vi "add_alignment_text.vi"(4 "Font, Size & Style":T1, 6 "Color":u32, 11 "image in":T2) -> (3 "image out":T2)   [LabVIEW 2011]
uses:
  <vilib>/vision/Image Controls.llb/IMAQ Image.ctl
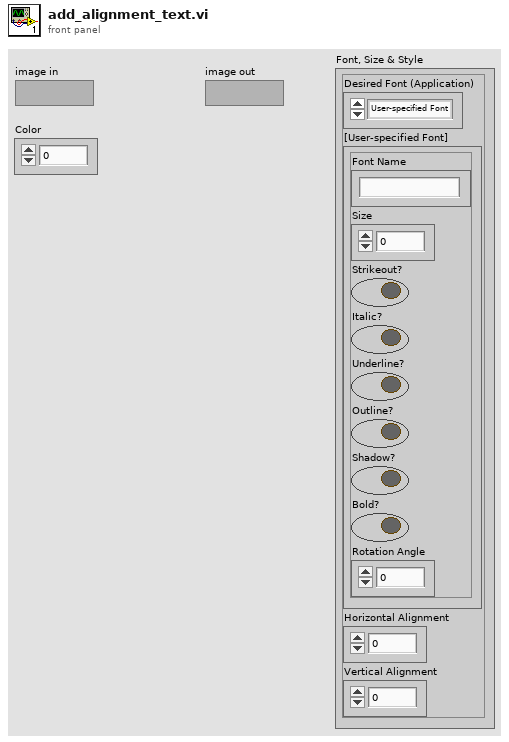
[diagram p1: front panel]
types:
  T1 = cluster{"Desired Font (Application)":enum16{"User-specified Font", "Application Font", "System Font", "Dialog Font"}, "[User-specified Font]":cluster{"Font Name":string, "Size":i16, "Strikeout?":bool, "Italic?":bool, "Underline?":bool, "Outline?":bool, "Shadow?":bool, "Bold?":bool, "Rotation Angle":dbl}, "Horizontal Alignment":i16, "Vertical Alignment":i16}
  T2 = typedef "IMAQ Image.ctl" = refnum<image>
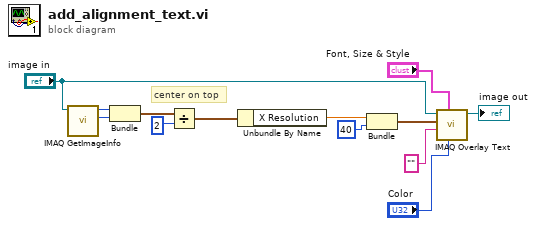
[diagram p0: block diagram]
diagram:
  # "center on top"
  n1 = call "IMAQ GetImageInfo"("Image"="image in") -> ("Y Resolution"=w3:i32, "X Resolution"=w4:i32)  [unwired: 3 in, 6 out]
  n2 = Bundle("X Resolution"=w4, "Y Resolution"=w3) -> (w1:cluster{"X Resolution":i32, "Y Resolution":i32})  [unwired: 1 in]
  n3 = Divide(x=w1, y=2 ("y height(Px)")) -> (x/y=w10:cluster{"X Resolution":dbl, "Y Resolution":dbl})
  n4 = Unbundle By Name(w10) -> ("X Resolution"=w11:dbl)
  n5 = Bundle("X Resolution"=w11, 40) -> (w5:cluster{"X Resolution":dbl, i32})  [unwired: 1 in]
  n6 = call "IMAQ Overlay Text"("Text Color (black)"="Color", "Font, Size & Style"="Font, Size & Style", "String"="", "Origin"=w5, "Image"="image in") -> ("Image Out"=→"image out":T2)  [unwired: 5 in, 1 out]
